vi "smff-simulate-motor.vi"(6 "Use Noise":bool, 8 "Time":dbl=-1.0, 11 "CO-ControlOutput":dbl) -> (3 "Motor Speed":dbl)   [LabVIEW 2019]
uses:
  <vilib>/Rock Robotics/WPI/ThirdParty/JAS_Junk/TrajLib/VI/TimeInterpDouble_New.vi
  <vilib>/Rock Robotics/WPI/ThirdParty/JAS_Junk/TrajLib/VI/TimeInterpDouble_AddSample.vi
  <vilib>/Rock Robotics/WPI/ThirdParty/JAS_Junk/TrajLib/VI/TimeInterpDouble_GetSample.vi
  <vilib>/Rock Robotics/WPI/ThirdParty/JAS_Junk/TrajLib/VI/TimeInterpDouble_SetMaxTime.vi
  <vilib>/Rock Robotics/WPI/ThirdParty/JAS_Junk/TrajLib/VI/TimeInterpDouble_CleanUp.vi
  <vilib>/Rock Robotics/WPI/ThirdParty/JAS_Junk/TrajLib/MathUtil_Interpolate.vi
  <vilib>/gmath/interp.llb/Search Ordered Table.vi
  <vilib>/Rock Robotics/WPI/ThirdParty/JAS_Junk/TrajLib/Trajectory_Library.lvlib
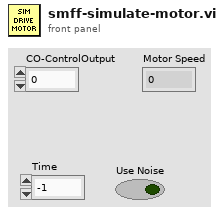
[diagram p1: front panel]
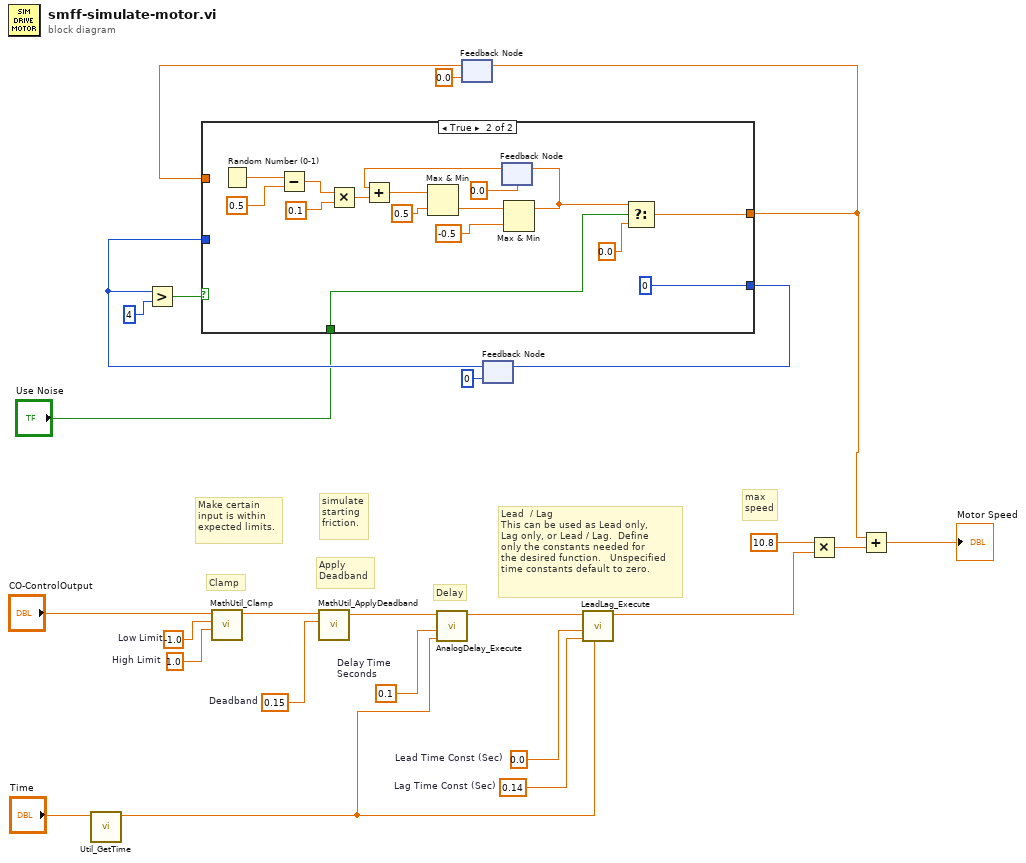
[diagram p0: block diagram]
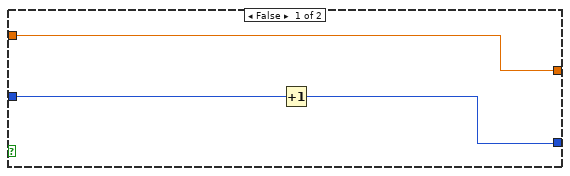
[diagram p2: hidden frame]
diagram:
  w6 = 0.14  # Lag Time Const (Sec)
  w5 = 0.0  # Lead Time Const (Sec)
  w8 = 0.1  # Delay Time Seconds
  w10 = 0.15  # Deadband
  w13 = 1.0  # High Limit
  w12 = -1.0  # Low Limit
  # "max \nspeed"
  # "simulate\nstarting\nfriction."
  # "Make certain\ninput is within\nexpected limits."
  # "Lead  / Lag\nThis can be used as Lead only, \nLag only, or Lead / Lag.  Define\nonly the constants needed for \nthe desired function.   Unspecified\ntime constants default to zero."
  # "Delay"
  # "Apply\nDeadband"
  # "Clamp"
  n1 = call <vilib>:"Util_GetTime.vi"("Pass_Through_Time"="Time") -> ("FPGA_Time_Seconds"=w1:dbl)  [unwired: 9 in, 1 out]
  n2 = call <vilib>:"MathUtil_Clamp.vi"("High Limit"=w13, "Low Limit"=w12, "Value"="CO-ControlOutput") -> ("Result"=w9:dbl)  [unwired: 8 in]
  n3 = call <vilib>:"MathUtil_ApplyDeadband.vi"("Deadband"=w10, "Value"=w9) -> ("Result"=w7:dbl)  [unwired: 9 in]
  n4 = call <vilib>:"AnalogDelay_Execute.vi"("Time"=w1, "Delay Time"=w8, "Input"=w7) -> ("Output"=w4:dbl)  [unwired: 7 in, 1 out]
  n5 = feedback #1(0.0 ("f")) -> (w15:dbl)
  n6 = feedback #2(0) -> (w18:i32)
  n7 = Greater?(x=w18, y=4) -> (0:w20:bool)
  n8 = case shown="True" w20 {
    tunnel: [w27 0] -> w22
    tunnel: w18 -> [w28 _]
    tunnel: [w26 w30] -> w17
    tunnel: w15 -> [w26 _]
    tunnel: "Use Noise" -> [_ w29]
    frame False {
      n9 = Increment(x=w28) -> (x+1=w27:i32)
    }
    frame True {
      n10 = Random Number (0-1)() -> (number: 0 to 1=w33:dbl)
      n11 = Subtract(x=w33, y=0.5) -> (x-y=w37:dbl)
      n12 = Multiply(x=w37, y=0.1) -> (x*y=w36:dbl)
      n13 = feedback #3(0.0) -> (w39:dbl)
      n14 = Add(x=w39, y=w36) -> (x+y=w43:dbl)
      n15 = Max & Min(x=w43, y=0.5) -> (min(x,y)=w42:dbl)  [unwired: 1 out]
      n16 = Max & Min(x=w42, y=-0.5) -> (max(x,y)=w34:dbl)  [unwired: 1 out]
      n17 = feedback-in #3(w34) -> ()
      n18 = Select(t=w34, s=w29, f=0.0) -> (s? t:f=w30:dbl)
    }
  }
  n19 = feedback-in #1(w17) -> ()
  n20 = feedback-in #2(w22) -> ()
  n21 = call <vilib>:"LeadLag_Execute.vi"("Time (Secs)"=w1, "Lag Time Const (Sec)"=w6, "Lead Time Const (Sec)"=w5, "Input"=w4) -> ("Output"=w3:dbl)  [unwired: 7 in]
  n22 = Multiply(x=10.8, y=w3) -> (x*y=w23:dbl)
  n23 = Add(x=w17, y=w23) -> (x+y=→"Motor Speed":dbl)
